vi "Convert LabVIEW Image Data To IMAQ.vi"(8 "error in (no error)":errorcluster, 10 "Image Data":T2, 11 "Image In":T1) -> (0 "error out":errorcluster, 3 "Image Out":T1)   [LabVIEW 2023]
doc: "This VI converts a LabVIEW Image into an IMAQ image."
uses:
  <vilib>/picture/picture.llb/imagedata.ctl
  <vilib>/vision/Image Controls.llb/IMAQ Image.ctl
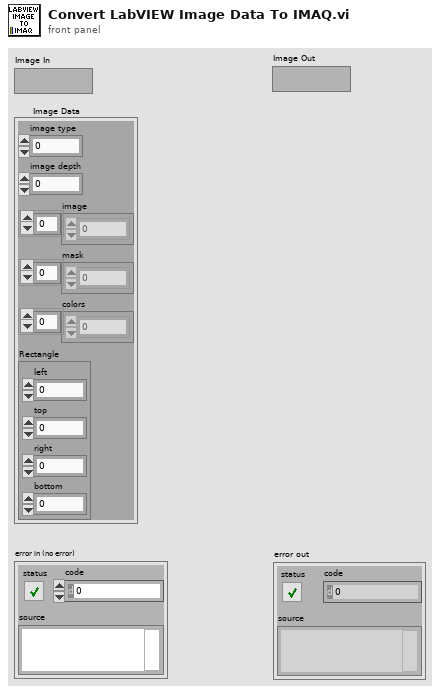
[diagram p1: front panel]
types:
  T1 = typedef "IMAQ Image.ctl" = refnum<image>
  T2 = typedef "imagedata.ctl" = cluster{"image type":i32, "image depth":i32, "image":u8[], "mask":u8[], "colors":u32[], "Rectangle":cluster{"left":i16, "top":i16, "right":i16, "bottom":i16}}
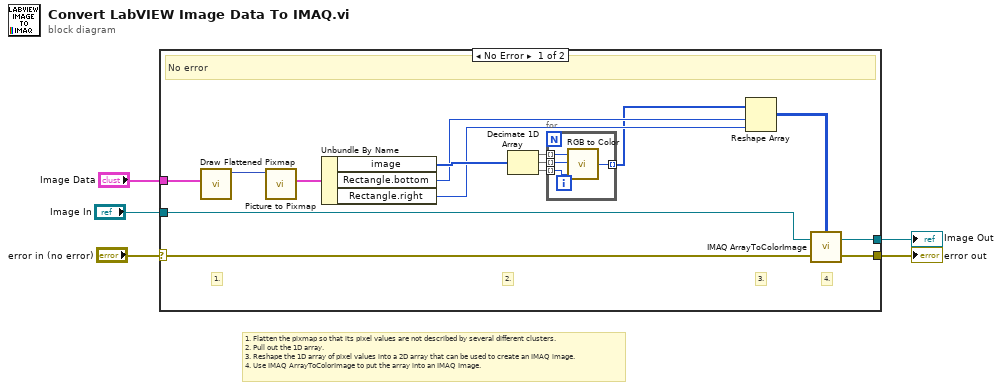
[diagram p0: block diagram]
diagram:
  # "1. Flatten the pixmap so that its pixel values are not described by several different clusters.\n2. Pull out the 1D array.\n3. Reshape the 1D array of pixel values into a 2D array that can be used to create an IMAQ image.\n4. Use IMAQ ArrayToColorImage to put the array into an IMAQ Image."
  n1 = case shown="No Error" "error in (no error)" {
    selector: "error in (no error)" -> [w6 w26]
    tunnel: [w14 w25] -> w5
    tunnel: [w13 w26] -> w4
    tunnel: "Image Data" -> [w12 _]
    tunnel: "Image In" -> [w11 w25]
    frame No Error {
      # "4."
      # "3."
      # "2."
      # "1."
      # "No error"
      n2 = call <vilib>:"Draw Flattened Pixmap.vi"("image data"=w12) -> ("new picture"=w20:picture)  [unwired: 8 in]
      n3 = call <vilib>:"Picture to Pixmap.vi"("picture"=w20) -> ("image data"=w19:T2)  [unwired: 9 in, 1 out]
      n4 = Unbundle By Name(w19) -> ("image"=w18:u8[], "Rectangle.bottom"=w17:i16, "Rectangle.right"=w16:i16)
      n5 = Decimate 1D Array(w18) -> (w10:u8[], w9:u8[], w8:u8[])
      n6 = for {
        tunnel: w10 -> [w24] mode=indexing
        tunnel: w9 -> [w23] mode=indexing
        tunnel: w8 -> [w22] mode=indexing
        tunnel: [w21] -> w7 mode=indexing
        n7 = call <vilib>:"RGB to Color.vi"("B"=w22, "G"=w23, "R"=w24) -> ("Color"=w21:u32)
      }
      n8 = Reshape Array(w7, w17, w16) -> (w15:u32[][])
      n9 = call "IMAQ ArrayToColorImage"("Image Pixels (U32)"=w15, "Image"=w11, "error in (no error)"=w6) -> ("Image Out"=w14:T1, "error out"=w13:errorcluster)  [unwired: 2 in]
    }
    frame Error {
      # "Error"
    }
  }
  "Image Out" <- w5
  "error out" <- w4
